vi "Dispose.vi"(8 "error in (no error)":errorcluster, 11 "Door":refnum<class "Door.lvclass">) -> (0 "error out":errorcluster)   [LabVIEW 2020, in "Door.lvclass"]
uses:
  Door.lvclass
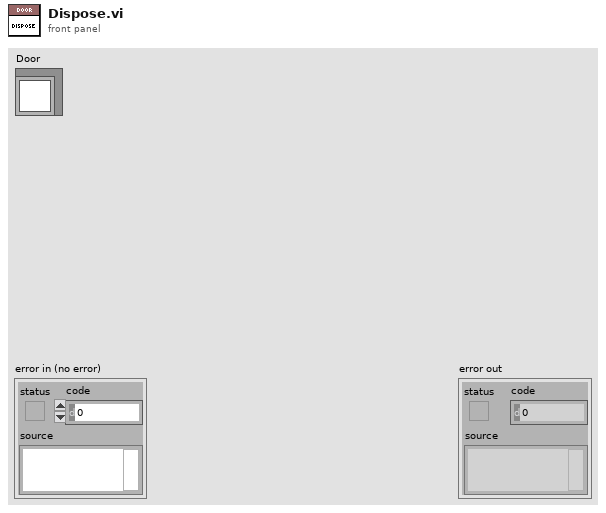
[diagram p1: front panel]
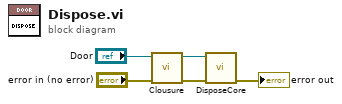
[diagram p0: block diagram]
diagram:
  n1 = call-dynamic "Clousure.vi"("error in (no error)"="error in (no error)", "Door"="Door") -> ("error out"=w1:errorcluster, "Door"=w2:refnum<class "Door.lvclass">)  [unwired: 8 in]
  n2 = call-dynamic "DisposeCore.vi"("error in (no error)"=w1, "Door"=w2) -> ("error out"=→"error out":errorcluster)  [unwired: 8 in, 1 out]
